vi "WriteRead.vi"(8 "error in (no error)":errorcluster, 10 "Command":string, 11 "Serial in":refnum<class "Serial.lvclass">) -> (0 "error out":errorcluster, 2 "Response":string, 3 "Serial out":refnum<class "Serial.lvclass">)   [LabVIEW 2014, in "Serial.lvclass"]
uses:
  Serial.lvclass
  Serial.lvclass/Serial.ctl
panel:
  out "Bytes Sent":u32
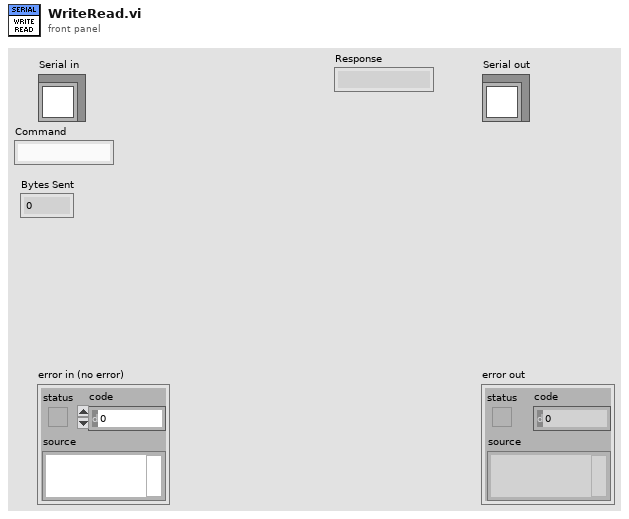
[diagram p1: front panel]
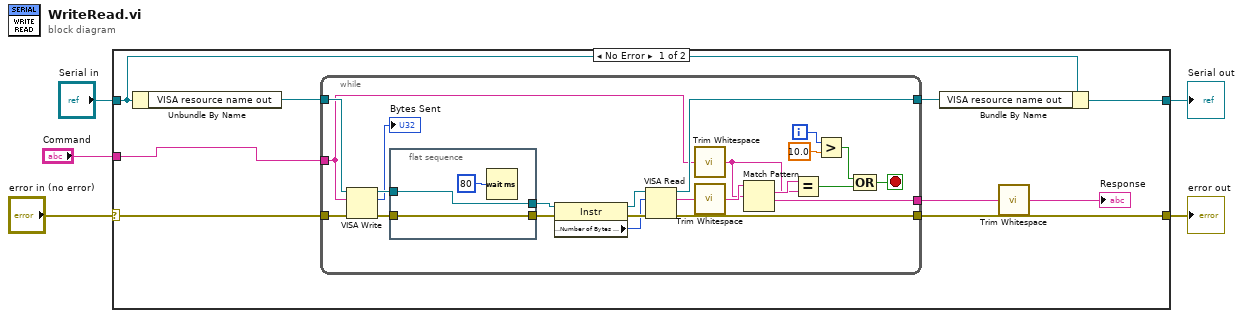
[diagram p0: block diagram]
diagram:
  n1 = case shown="No Error" "error in (no error)" {
    selector: "error in (no error)" -> [w13 w42]
    tunnel: [w12 w42] -> w4
    tunnel: [w10 w41] -> w2
    tunnel: "Serial in" -> [w11 w41]
    tunnel: "Command" -> [w6 _]
    frame No Error {
      n2 = Unbundle By Name(w11) -> ("VISA resource name out"=w14:refnum<visa-resource-name>)
      n3 = while {
        tunnel: w14 -> [w37]
        tunnel: w13 -> [w36]
        tunnel: [w35] -> w9
        tunnel: [w34] -> w12
        tunnel: w6 -> [w22]
        tunnel: [w30] -> w8
        i -> [w20]
        stop <- w17 stop-if-true
        n4 = VISA Write(VISA resource name=w37, write buffer=w22, error in (no error)=w36) -> (VISA resource name out=w28:refnum<visa-resource-name>, return count=→"Bytes Sent":u32, error out=w25:errorcluster)
        n5 = flat-sequence {
          tunnel: [w40] -> w27
          tunnel: w28 -> [w40]
          tunnel: w25 -> [w39]
          tunnel: [w39] -> w26
          frame #0 {
            n6 = Wait (ms)(milliseconds to wait=u32 80) -> ()  [unwired: 1 out]
          }
        }
        n7 = property class="Instr"(reference=w27, error in=w26) -> (reference out=w33:refnum<visa-resource-name>, error out=w32:errorcluster, "Serial Settings:Number of Bytes at Serial Port"=w31:u32)
        n8 = VISA Read(VISA resource name=w33, byte count=w31, error in (no error)=w32) -> (VISA resource name out=w35:refnum<visa-resource-name>, read buffer=w24:string, error out=w34:errorcluster)  [unwired: 1 out]
        n9 = call <vilib>:"Trim Whitespace.vi"("string"=w22) -> ("trimmed string"=w16:string)  [unwired: 1 in]
        n10 = call <vilib>:"Trim Whitespace.vi"("string"=w24) -> ("trimmed string"=w23:string)  [unwired: 1 in]
        n11 = Match Pattern(string=w23, regular expression=w16) -> (match substring=w29:string, after substring=w30:string)  [unwired: 1 in, 2 out]
        n12 = Equal?(x=w29, y=w16) -> (x = y?=w18:bool)
        n13 = Greater?(x=w20, y=10.0) -> (0:w19:bool)
        n14 = Compound Arithmetic op=OR(w19, w18) -> (w17:bool)
      }
      n15 = Bundle By Name(cluster=w11, "VISA resource name out"=w9) -> (w10:refnum<class "Serial.lvclass">)
      n16 = call <vilib>:"Trim Whitespace.vi"("string"=w8) -> ("trimmed string"=→"Response":string)  [unwired: 1 in]
    }
    frame Error {
    }
  }
  "error out" <- w4
  "Serial out" <- w2
